vi "Push Ptr Back to CacheQueue.vi"(8 "error in":errorcluster, 10 "Cache Length":i32, 11 "MDPtr DVR":refnum<data-value>) -> (0 "error out":errorcluster)   [LabVIEW 2017, in "MDPtr.lvlib" / "MDPtrMgr.lvclass"]
uses:
  MDPtrMgr.lvclass
  MDPtr TypeDef/MDPtr DataFrame-Memory.ctl
  MDPtr TypeDef/MDPtr DataFrame-Common.ctl
  <vilib>/Utility/Data Type/Type Definitions/Data Type.ctl
  MDPtr.lvlib
  <vilib>/Utility/Data Type/NI_Data Type.lvlib
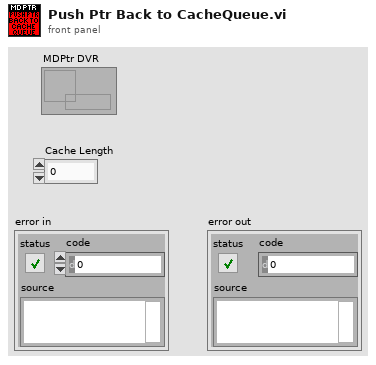
[diagram p1: front panel]
types:
  T1 = typedef "MDPtr.lvlib/MDPtr Queue.ctl" = refnum<queue>
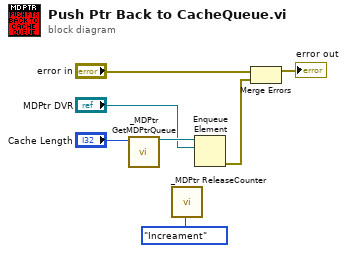
[diagram p0: block diagram]
diagram:
  n1 = call "_MDPtr GetMDPtrQueue.vi"("MemoryLength"="Cache Length") -> ("MDPtrQueue"=w6:T1)  [unwired: 8 in, 2 out]
  n2 = call "_MDPtr ReleaseCounter.vi"("Oper(Get)"=enum16{"GET", "Increament", "decreament"}."Increament") -> ()  [unwired: 9 in, 2 out]
  n3 = Enqueue Element(queue=w6, element="MDPtr DVR") -> (error out=w3:errorcluster)  [unwired: 2 in, 2 out]
  n4 = Merge Errors("error in", w3) -> (→"error out":errorcluster)
